vi "Override Calibrations + Settings 2016.vi"   [LabVIEW 2015]
uses:
  Global Variables/Settings.vi
  Global Variables/Calibrations.vi
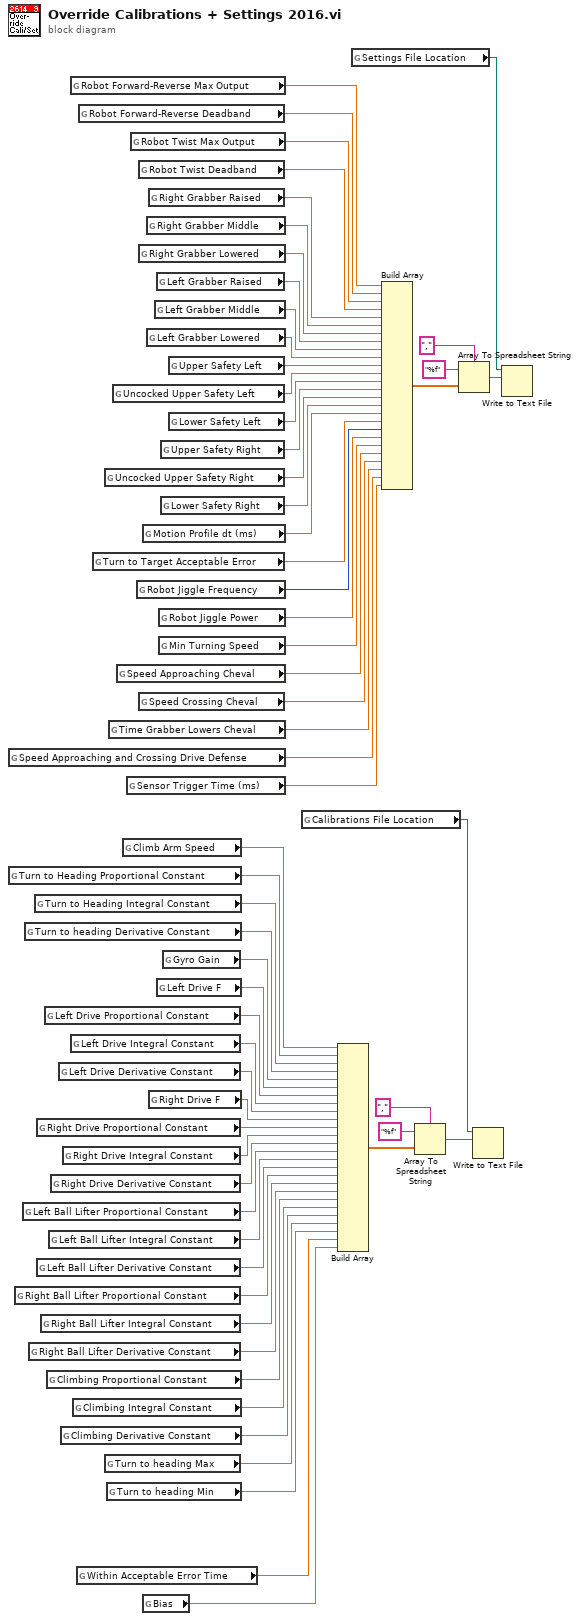
[diagram p0: block diagram]
diagram:
  n1 = global read "Settings.vi" "Speed Approaching and Crossing Drive Defense"() -> (w4:dbl)
  n2 = global read "Calibrations.vi" "Turn to Heading Proportional Constant"() -> (w17:dbl)
  n3 = global read "Calibrations.vi" "Right Ball Lifter Proportional Constant"() -> (w30:dbl)
  n4 = global read "Calibrations.vi" "Left Ball Lifter Proportional Constant"() -> (w27:dbl)
  n5 = global read "Calibrations.vi" "Turn to heading Derivative Constant"() -> (w18:dbl)
  n6 = global read "Calibrations.vi" "Right Ball Lifter Derivative Constant"() -> (w32:dbl)
  n7 = global read "Calibrations.vi" "Turn to Heading Integral Constant"() -> (w11:dbl)
  n8 = global read "Calibrations.vi" "Right Drive Proportional Constant"() -> (w24:dbl)
  n9 = global read "Calibrations.vi" "Left Ball Lifter Derivative Constant"() -> (w29:dbl)
  n10 = global read "Calibrations.vi" "Right Ball Lifter Integral Constant"() -> (w31:dbl)
  n11 = global read "Calibrations.vi" "Left Drive Proportional Constant"() -> (w21:dbl)
  n12 = global read "Calibrations.vi" "Climbing Proportional Constant"() -> (w14:dbl)
  n13 = global read "Calibrations.vi" "Left Ball Lifter Integral Constant"() -> (w28:dbl)
  n14 = global read "Calibrations.vi" "Right Drive Derivative Constant"() -> (w26:dbl)
  n15 = global read "Calibrations.vi" "Left Drive Derivative Constant"() -> (w13:dbl)
  n16 = global read "Calibrations.vi" "Climbing Derivative Constant"() -> (w16:dbl)
  n17 = global read "Calibrations.vi" "Right Drive Integral Constant"() -> (w25:dbl)
  n18 = global read "Settings.vi" "Robot Forward-Reverse Max Output"() -> (w43:dbl)
  n19 = global read "Calibrations.vi" "Left Drive Integral Constant"() -> (w22:dbl)
  n20 = global read "Calibrations.vi" "Climbing Integral Constant"() -> (w15:dbl)
  n21 = global read "Calibrations.vi" "Within Acceptable Error Time"() -> (w2:dbl)
  n22 = global read "Settings.vi" "Robot Forward-Reverse Deadband"() -> (w42:dbl)
  n23 = global read "Settings.vi" "Turn to Target Acceptable Error"() -> (w37:dbl)
  n24 = global read "Settings.vi" "Uncocked Upper Safety Right"() -> (w50:dbl)
  n25 = global read "Calibrations.vi" "Turn to heading Max"() -> (w10:dbl)
  n26 = global read "Calibrations.vi" "Turn to heading Min"() -> (w9:dbl)
  n27 = global read "Settings.vi" "Time Grabber Lowers Cheval"() -> (w5:dbl)
  n28 = global read "Settings.vi" "Uncocked Upper Safety Left"() -> (w41:dbl)
  n29 = global read "Settings.vi" "Speed Approaching Cheval"() -> (w7:dbl)
  n30 = global read "Calibrations.vi" "Climb Arm Speed"() -> (w23:dbl)
  n31 = global read "Settings.vi" "Sensor Trigger Time (ms)"() -> (w3:dbl)
  n32 = global read "Settings.vi" "Robot Twist Max Output"() -> (w44:dbl)
  n33 = global read "Settings.vi" "Robot Jiggle Frequency"() -> (w35:i32)
  n34 = global read "Settings.vi" "Robot Twist Deadband"() -> (w38:dbl)
  n35 = global read "Settings.vi" "Right Grabber Lowered"() -> (w47:dbl)
  n36 = global read "Settings.vi" "Speed Crossing Cheval"() -> (w6:dbl)
  n37 = global read "Settings.vi" "Motion Profile dt (ms)"() -> (w48:dbl)
  n38 = global read "Calibrations.vi" "Bias"() -> (w1:dbl)
  n39 = global read "Settings.vi" "Right Grabber Middle"() -> (w46:dbl)
  n40 = global read "Settings.vi" "Left Grabber Lowered"() -> (w39:dbl)
  n41 = global read "Settings.vi" "Right Grabber Raised"() -> (w45:dbl)
  n42 = global read "Calibrations.vi" "Right Drive F"() -> (w12:dbl)
  n43 = global read "Settings.vi" "Left Grabber Middle"() -> (w53:dbl)
  n44 = global read "Settings.vi" "Left Grabber Raised"() -> (w54:dbl)
  n45 = global read "Calibrations.vi" "Left Drive F"() -> (w20:dbl)
  n46 = global read "Settings.vi" "Robot Jiggle Power"() -> (w36:dbl)
  n47 = global read "Settings.vi" "Min Turning Speed"() -> (w33:dbl)
  n48 = global read "Settings.vi" "Upper Safety Right"() -> (w51:dbl)
  n49 = global read "Settings.vi" "Lower Safety Right"() -> (w49:dbl)
  n50 = global read "Calibrations.vi" "Gyro Gain"() -> (w19:dbl)
  n51 = global read "Settings.vi" "Upper Safety Left"() -> (w40:dbl)
  n52 = global read "Settings.vi" "Lower Safety Left"() -> (w52:dbl)
  n53 = global read "Calibrations.vi" "Calibrations File Location"() -> (w55:path)
  n54 = Build Array(w23, w17, w11, w18, w19, w20, w21, w22, w13, w12, w24, w25, w26, w27, w28, w29, w30, w31, w32, w14, w15, w16, w10, w9, w2, w1) -> (w8:dbl[])
  n55 = global read "Settings.vi" "Settings File Location"() -> (w56:path)
  n56 = Build Array(w43, w42, w44, w38, w45, w46, w47, w54, w53, w39, w40, w41, w52, w51, w50, w49, w48, w37, w35, w36, w33, w7, w6, w5, w4, w3) -> (w34:dbl[])
  n57 = Array To Spreadsheet String(delimiter (Tab)=",", array=w8, 3:"%f" ("format string")) -> (spreadsheet string=w57:string)
  n58 = Array To Spreadsheet String(delimiter (Tab)=",", array=w34, 3:"%f" ("format string")) -> (spreadsheet string=w60:string)
  n59 = Write to Text File(file (use dialog)=w55, text=w57) -> ()  [unwired: 2 in, 3 out]
  n60 = Write to Text File(file (use dialog)=w56, text=w60) -> ()  [unwired: 2 in, 3 out]
